vi "Plugin Configuration.Set Transfer Group Configurations.vi"(10 "Transfer Group Configurations":refnum<class "Transfer Group Configuration.lvclass">[](array[class]), 11 "Plugin Configuration in":refnum<class "Plugin Configuration.lvclass">) -> (3 "Plugin Configuration out":refnum<class "Plugin Configuration.lvclass">)   [LabVIEW 2017, in "DSF Core.lvlib" / "Plugin Configuration.lvclass"]
uses:
  Plugin Configuration.lvclass
  Transfer Group/Transfer Group Configuration.lvclass
  Plugin Configuration.lvclass/Plugin Configuration.ctl
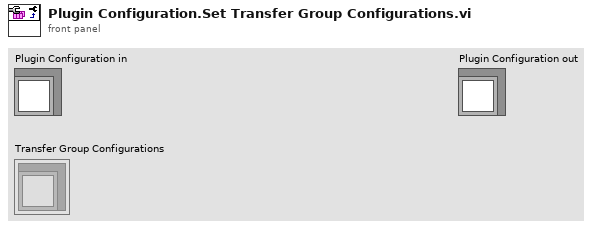
[diagram p1: front panel]
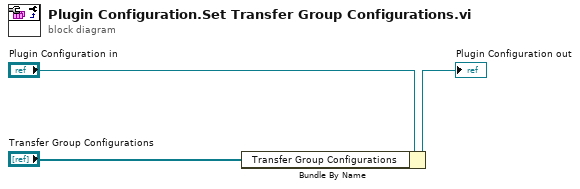
[diagram p0: block diagram]
diagram:
  n1 = Bundle By Name(cluster="Plugin Configuration in", "Transfer Group Configurations"="Transfer Group Configurations") -> (→"Plugin Configuration out":refnum<class "Plugin Configuration.lvclass">)
